vi "Set Field_not used.vi"(6 "Positive?":bool, 7 "VISA session":refnum<visa-resource-name>, 8 "error in (no error)":errorcluster, 9 "Desired Field":dbl, 10 "Voltage Limit":dbl=2255.0 format="%.2f", 11 "input cluster":T1) -> (0 "error out":errorcluster, 3 "output cluster":T1, 5 "dup VISA session":refnum<visa-resource-name>)   [LabVIEW 2012]
uses:
  Magna Power Constants.vi
  <vilib>/gmath/NI_Gmath.lvlib
panel:
  out "Actual field":dbl
  out "Current guess":dbl
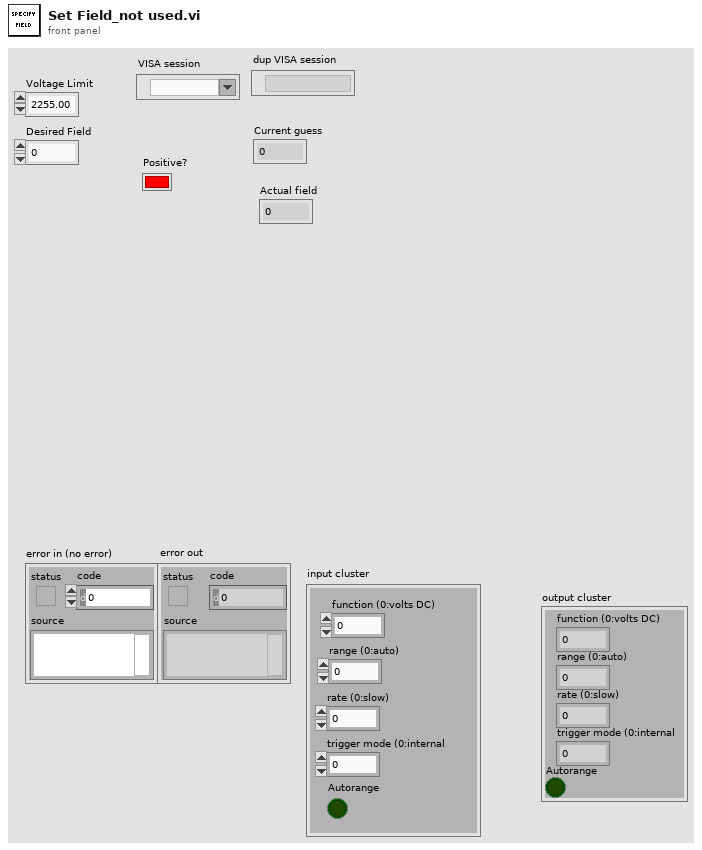
[diagram p1: front panel]
types:
  T1 = cluster{"function (0:volts DC)":i16, "range (0:auto)":i16, "rate (0:slow)":i16, "trigger mode (0:internal":i16, "Autorange":bool}
  T2 = cluster{"Magna Current":dbl[], "Magnetic Field":dbl[], "Fluke Voltage":dbl[]}
  T3 = cluster{"Field":dbl[], "Current Derivative":dbl[]}
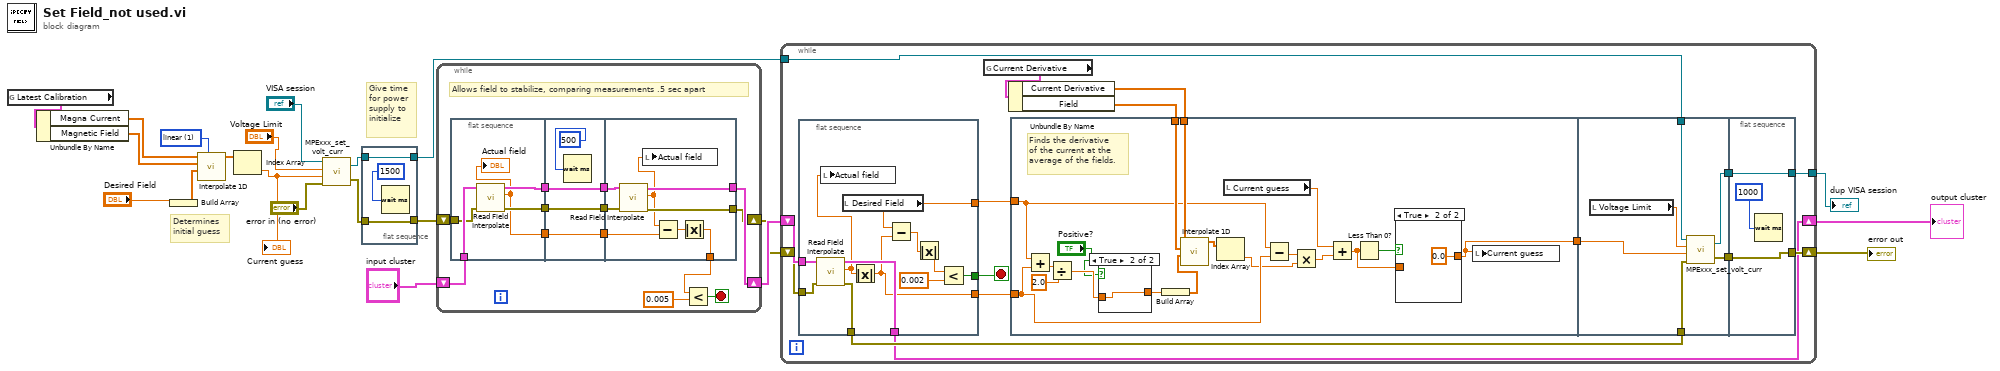
[diagram p0: block diagram]
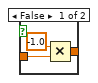
[diagram p3: hidden frame]
diagram:
  w20 = 1 items=["nearest", "linear", "spline", "cubic Hermite", "Lagrange"] ("method")
  # "Give time\nfor power\nsupply to\ninitialize"
  # "Determines\ninitial guess"
  n1 = global read "Magna Power Constants.vi" "Latest Calibration"() -> (w21:T2)
  n2 = Unbundle By Name(w21) -> ("Magna Current"=w12:dbl[], "Magnetic Field"=w13:dbl[])
  n3 = Build Array("Desired Field") -> (w19:dbl[])
  n4 = call <vilib>:"Interpolate 1D.vi"("method"=w20, "xi"=w19, "X"=w13, "Y"=w12) -> ("yi"=w18:dbl[])  [unwired: 5 in, 2 out]
  n5 = Index Array(array=w18) -> (element=w17:dbl)  [unwired: 1 in]
  "Current guess" <- w17
  n6 = call "MPExxx_set_volt_curr.vi"("error in (no error)"="error in (no error)", "Set Current"=w17, "Set Voltage"="Voltage Limit", "VISA session"="VISA session") -> ("error out"=w16:errorcluster, "dup VISA session"=w15:refnum<visa-resource-name>)
  n7 = flat-sequence {
    tunnel: [w23] -> w8
    tunnel: w16 -> [w23]
    tunnel: w15 -> [w22]
    tunnel: [w22] -> w5
    frame #0 {
      n8 = Wait (ms)(milliseconds to wait=u32 1500) -> ()  [unwired: 1 out]
    }
  }
  n9 = while {
    shift-right: [w28] -> w7
    shift-left: "input cluster" -> [w37]
    shift-right: [w26] -> w6
    shift-left: w8 -> [w36]
    stop <- w31 stop-if-true
    # "Allows field to stabilize, comparing measurements .5 sec apart"
    n10 = flat-sequence {
      tunnel: w37 -> [w42]
      tunnel: w36 -> [w41]
      tunnel: [w40] -> w34
      tunnel: [w39] -> w32
      tunnel: [w38] -> w29
      tunnel: [w44] -> w35
      tunnel: w34 -> [w44]
      tunnel: [w45] -> w33
      tunnel: w32 -> [w45]
      tunnel: [w43] -> w30
      tunnel: w29 -> [w43]
      tunnel: w35 -> [w54]
      tunnel: w33 -> [w53]
      tunnel: w30 -> [w51]
      tunnel: [w50] -> w28
      tunnel: [w49] -> w25
      tunnel: [w48] -> w26
      frame #0 {
        n11 = call "Read Field Interpolate.vi"("error in (no error)"=w41, "input cluster"=w42) -> ("error out"=w39:errorcluster, "Field (T)"=w38:dbl, "output cluster"=w40:T1)  [unwired: 4 in, 3 out]
        "Actual field" <- w38
      }
      frame #1 {
        n12 = Wait (ms)(milliseconds to wait=u32 500) -> ()  [unwired: 1 out]
      }
      frame #2 {
        n13 = call "Read Field Interpolate.vi"("error in (no error)"=w53, "input cluster"=w54) -> ("error out"=w48:errorcluster, "Field (T)"=w47:dbl, "output cluster"=w50:T1)  [unwired: 4 in, 3 out]
        n14 = local write "Actual field"(w47) -> ()
        n15 = Subtract(x=w47, y=w51) -> (x-y=w52:dbl)
        n16 = Absolute Value(x=w52) -> (abs(x)=w49:dbl)
      }
    }
    n17 = Less?(x=w25, y=0.005) -> (x < y?=w31:bool)
  }
  n18 = while {
    tunnel: w5 -> [w62]
    shift-right: [w59] -> w3
    shift-left: w6 -> [w69]
    tunnel: [w57] -> w2
    shift-right: [w55] -> w1
    shift-left: w7 -> [w70]
    stop <- w68 stop-if-true
    n19 = flat-sequence {
      tunnel: w70 -> [w114]
      tunnel: w69 -> [w113]
      tunnel: [w111] -> w68
      tunnel: [w105] -> w64
      tunnel: [w108] -> w63
      tunnel: [w107] -> w61
      tunnel: [w106] -> w55
      frame #0 {
        n20 = call "Read Field Interpolate.vi"("error in (no error)"=w113, "input cluster"=w114) -> ("error out"=w107:errorcluster, "Field (T)"=w104:dbl, "output cluster"=w106:T1)  [unwired: 4 in, 3 out]
        n21 = local write "Actual field"(w104) -> ()
        n22 = local read "Desired Field"() -> (w108:dbl)
        n23 = Absolute Value(x=w104) -> (abs(x)=w105:dbl)
        n24 = Subtract(x=w108, y=w105) -> (x-y=w110:dbl)
        n25 = Absolute Value(x=w110) -> (abs(x)=w109:dbl)
        n26 = Less?(x=w109, y=0.002) -> (x < y?=w111:bool)
      }
    }
    n27 = global read "Magna Power Constants.vi" "Current Derivative"() -> (w65:T3)
    n28 = Unbundle By Name(w65) -> ("Current Derivative"=w66:dbl[], "Field"=w67:dbl[])
    n29 = flat-sequence {
      tunnel: w67 -> [w86]
      tunnel: w66 -> [w85]
      tunnel: w64 -> [w78]
      tunnel: w63 -> [w79]
      tunnel: [w72] -> w60
      tunnel: w62 -> [w100]
      tunnel: w61 -> [w99]
      tunnel: w60 -> [w97]
      tunnel: [w96] -> w58
      tunnel: [w95] -> w56
      tunnel: [w102] -> w59
      tunnel: w58 -> [w102]
      tunnel: [w101] -> w57
      tunnel: w56 -> [w101]
      frame #0 {
        # "Finds the derivative\nof the current at the\naverage of the fields."
        n30 = Add(x=w79, y=w78) -> (x+y=w83:dbl)
        n31 = Divide(x=w83, y=2.0) -> (x/y=w81:dbl)
        n32 = case shown="True" "Positive?" {
          tunnel: w81 -> [w92 w94]
          tunnel: [w91 w94] -> w88
          frame False {
            n33 = Multiply(x=-1.0, y=w92) -> (x*y=w91:dbl)
          }
          frame True {
          }
        }
        n34 = Build Array(w88) -> (w87:dbl[])
        n35 = call <vilib>:"Interpolate 1D.vi"("xi"=w87, "X"=w86, "Y"=w85) -> ("yi"=w84:dbl[])  [unwired: 6 in, 2 out]
        n36 = Index Array(array=w84) -> (element=w76:dbl)  [unwired: 1 in]
        n37 = local read "Current guess"() -> (w75:dbl)
        n38 = Subtract(x=w79, y=w78) -> (x-y=w77:dbl)
        n39 = Multiply(x=w77, y=w76) -> (x*y=w74:dbl)
        n40 = Add(x=w75, y=w74) -> (x+y=w71:dbl)
        n41 = Less Than 0?(x=w71) -> (x < 0?=w73:bool)
        n42 = case shown="True" w73 {
          tunnel: [w89 0.0] -> w72
          tunnel: w71 -> [w89 _]
          frame False {
          }
          frame True {
          }
        }
        n43 = local write "Current guess"(w72) -> ()
      }
      frame #1 {
        n44 = local read "Voltage Limit"() -> (w98:dbl)
        n45 = call "MPExxx_set_volt_curr.vi"("error in (no error)"=w99, "Set Current"=w97, "Set Voltage"=w98, "VISA session"=w100) -> ("error out"=w96:errorcluster, "dup VISA session"=w95:refnum<visa-resource-name>)
      }
      frame #2 {
        n46 = Wait (ms)(milliseconds to wait=u32 1000) -> ()  [unwired: 1 out]
      }
    }
  }
  "error out" <- w3
  "output cluster" <- w1
  "dup VISA session" <- w2
